vi "benchmark-jitter-tl.vi"(11 "iterations":i32=1000000) -> ()   [LabVIEW 2020]
uses:
  <vilib>/Platform/TimedLoop/XDataNode/timing_clust.ctl
  <vilib>/Platform/TimedLoop/XDataNode/nitl_modes.ctl
  <vilib>/Platform/TimedLoop/XDataNode/wakeup.ctl
  <vilib>/platform/TimedLoop/XDataNode/XDataNode.xnode
  <vilib>/Platform/TimedLoop/XDataNode/XDNodeRunTimeDep.lvlib
panel:
  in  "Period (ms)":i64
  out "wfmg":dbl[][](graph)
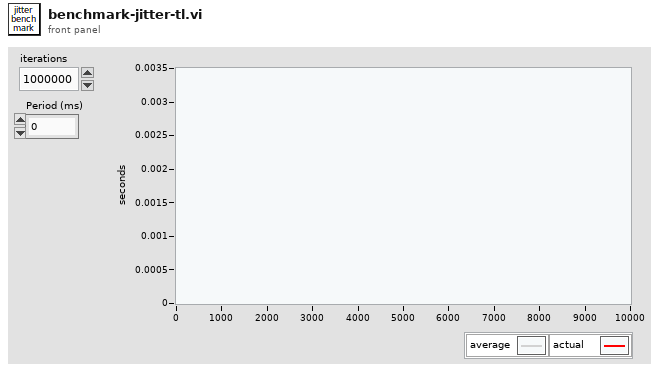
[diagram p1: front panel]
types:
  T1 = typedef "XDNodeRunTimeDep.lvlib/timing_clust.ctl" = cluster{"Expected End [f-1]":u64, "Actual End [f-1]":u64, "Finished Late? [f-1]":bool, "Expected End [i-1]":u64, "Actual End [i-1]":u64, "Finished Late? [i-1]":bool, "Expected Start [i]":u64, "Actual Start [i]":u64, "Expected Start [f]":u64, "Actual Start [f]":u64, "Source Name":string, "Structure Name":string, "Period":i64, "Deadline":i64, "Offset":i64, "Start":i64, "Priority":i32, "Timeout":i32, "Mode":T2, "Wakeup Reason":T3, "Error":errorcluster, "Source Type":string, "Secondary Source Type":string, "Global End Time":u64, "Global Start Time":u64, "Frame Duration":u64, "Iteration Duration":u64, "Assigned CPU":i32, "I/O Scan Engine Mode":u32}
  T2 = typedef "XDNodeRunTimeDep.lvlib/nitl_modes.ctl" = enum32{"No Change", "Process missed periods, maintain original phase", "Discard missed periods, maintain original phase", "Process missed periods, ignore original phase", "Discard missed periods, ignore original phase"}
  T3 = typedef "XDNodeRunTimeDep.lvlib/wakeup.ctl" = enum32{"Normal", "Aborted", "Asynchronous wakeup", "Timing source error", "Timed loop error", "Timeout"}
  T4 = typedef "metadata.ctl" = cluster{"worker ID":u32, "min (s)":dbl, "max (s)":dbl, "mean (s)":dbl, "duration (s)":dbl}
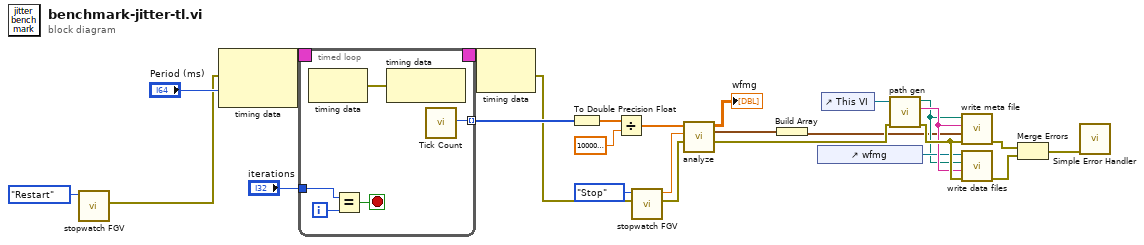
[diagram p0: block diagram]
diagram:
  n1 = call "stopwatch FGV.vi"("state"=enum16{"Restart", "Stop"}."Restart") -> ("error out"=w2:errorcluster)  [unwired: 9 in, 1 out]
  n2 = node-c288(w2, "Period (ms)") -> (w6:T1)
  n3 = timed-loop {
    tunnel: [w31] -> w9 mode=indexing
    timing: w6 -> [_]
    timing-out: [_] -> w5
    tunnel: "iterations" -> [w29]
    i -> [w30]
    stop <- w28 stop-if-true
    n4 = node-c288() -> (w27:errorcluster)  [unwired: 1 in]
    n5 = Equal?(x=w29, y=w30) -> (x = y?=w28:bool)
    n6 = node-c288(w27) -> ()  [unwired: 1 out]
    n7 = call "Tick Count"() -> ("Tick Count(uSec)"=w31:u32)
  }
  n8 = node-c288(w5) -> (w1:errorcluster)
  n9 = To Double Precision Float(number=w9) -> (double precision float=w8:dbl[])
  n10 = Divide(x=w8, y=1000000.0) -> (x/y=w21:dbl[])
  n11 = call "stopwatch FGV.vi"("error in"=w1, "state"=enum16{"Restart", "Stop"}."Stop") -> ("error out"=w19:errorcluster, "duration (s)"=w20:dbl)  [unwired: 8 in]
  n12 = call "analyze.vi"("error in"=w19, "duration (s)"=w20, "relative seconds"=w21) -> ("error out"=w24:errorcluster, "metadata"=w11:T4, "data"=→"wfmg":dbl[][])  [unwired: 6 in]
  n13 = Build Array(w11) -> (w10:T4[])
  n14 = control-ref of="wfmg"() -> (w15:refnum<vi>)
  n15 = control-ref of="This VI"() -> (w17:refnum<vi>)
  n16 = call "path gen.vi"("error in"=w24, "Calling VI"=w17) -> ("error out"=w18:errorcluster, "basename"=w16:string, "output folder"=w12:path)  [unwired: 7 in]
  n17 = call "write meta file.vi"("error in"=w18, "metadata"=w10, "file basename"=w16, "output folder"=w12) -> ("error out"=w14:errorcluster)  [unwired: 7 in]
  n18 = call "write data files.vi"("error in"=w18, "file basename"=w16, "output folder"=w12, "WaveformGraph in"=w15) -> ("error out"=w13:errorcluster)  [unwired: 7 in]
  n19 = Merge Errors(w14, w13) -> (w22:errorcluster)
  n20 = call <vilib>:"Simple Error Handler.vi"("error in (no error)"=w22) -> ()  [unwired: 4 in, 5 out]
